vi "Mysql data reader Scalar string.vi"(8 "error in (no error)":errorcluster, 11 ".NET Refnum in":refnum<k24>) -> (0 "error out":errorcluster, 3 "GetString":string)   [LabVIEW 2020, in "mysql.lvlib" / "mysql.lvclass"]
uses:
  mysql.lvclass
  MySql.Data
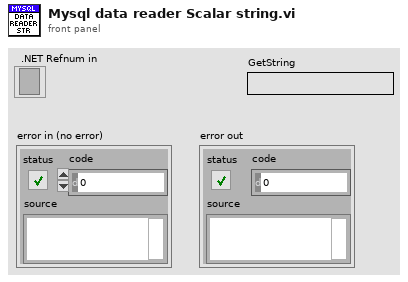
[diagram p1: front panel]
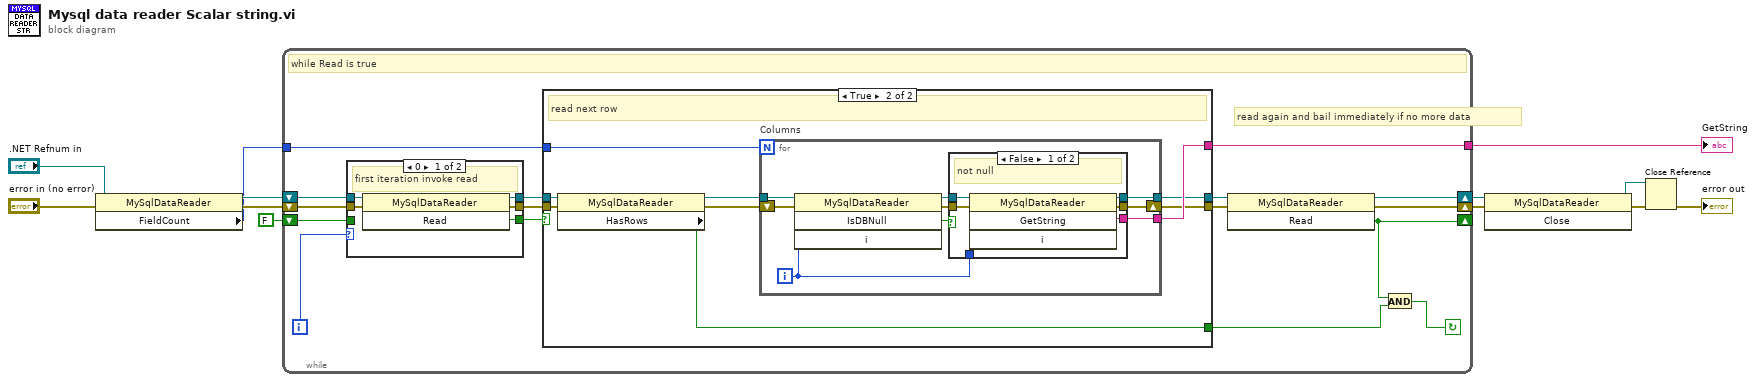
[diagram p0: block diagram]
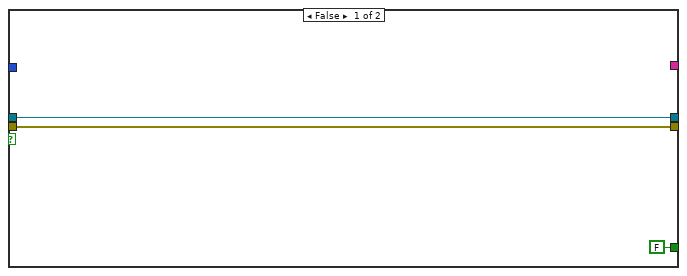
[diagram p3: hidden frame]
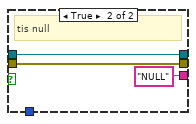
[diagram p4: hidden frame]
diagram:
  n1 = property class="MySqlDataReader"(reference=".NET Refnum in", error in="error in (no error)") -> (reference out=w8:refnum<k24>, error out=w7:errorcluster, "FieldCount"=w4:i32)
  n2 = while {
    tunnel: w4 -> [w28]
    tunnel: [w27] -> w5
    shift-right: [w21] -> w10
    shift-left: w7 -> [w26]
    shift-right: [w19] -> w9
    shift-left: w8 -> [w24]
    shift-right: [w14] -> _
    shift-left: FALSE ("Read") -> [w13]
    i -> [w15]
    stop <- w17 continue-if-true
    # "read again and bail immediately if no more data"
    # "while Read is true"
    n3 = case shown="0" w15 {
      tunnel: w26 -> [w33 w35]
      tunnel: [w32 w35] -> w25
      tunnel: w24 -> [w31 w36]
      tunnel: [w30 w36] -> w23
      tunnel: [w29 w34] -> w22
      tunnel: w13 -> [_ w34]
      frame 0 {
        # "first iteration invoke read"
        n4 = invoke class="MySqlDataReader" method="Read"(reference=w31, error in=w33) -> (reference out=w30:refnum<k24>, error out=w32:errorcluster, "Read"=w29:bool)  [unwired: 1 in]
      }
      frame 1.., Default {
        # "read after for other iterations"
      }
    }
    n5 = case shown="True" w22 {
      tunnel: w28 -> [_ w48]
      tunnel: [_ w47] -> w27
      tunnel: w25 -> [w38 w46]
      tunnel: w23 -> [w39 w45]
      tunnel: [w39 w44] -> w18
      tunnel: [w38 w40] -> w20
      tunnel: [FALSE ("HasRows") w41] -> w16
      frame False {
      }
      frame True {
        # "read next row"
        n6 = property class="MySqlDataReader"(reference=w45, error in=w46) -> (reference out=w43:refnum<k24>, error out=w42:errorcluster, "HasRows"=w41:bool)
        n7 = for "Columns" {
          N: w48 -> [_]
          tunnel: w43 -> [w52]
          shift-right: [w57] -> w40
          shift-left: w42 -> [w53]
          tunnel: [w56] -> w47
          tunnel: [w55] -> w44
          i -> [w54]
          n8 = invoke class="MySqlDataReader" method="IsDBNull"(reference=w52, error in=w53, "i"=w54) -> (reference out=w51:refnum<k24>, error out=w50:errorcluster, "IsDBNull"=w49:bool)  [unwired: 1 in, 1 out]
          n9 = case shown="False" w49 {
            tunnel: [w63 w65] -> w57
            tunnel: [w62 "NULL" ("GetString")] -> w56
            tunnel: [w61 w66] -> w55
            tunnel: w54 -> [w60 _]
            tunnel: w51 -> [w59 w66]
            tunnel: w50 -> [w58 w65]
            frame False {
              # "not null"
              n10 = invoke class="MySqlDataReader" method="GetString"(reference=w59, error in=w58, "i"=w60) -> (reference out=w61:refnum<k24>, error out=w63:errorcluster, "GetString"=w62:string)  [unwired: 1 in, 1 out]
            }
            frame True {
              # "tis null"
            }
          }
        }
      }
    }
    n11 = invoke class="MySqlDataReader" method="Read"(reference=w18, error in=w20) -> (reference out=w19:refnum<k24>, error out=w21:errorcluster, "Read"=w14:bool)  [unwired: 1 in]
    n12 = And(x=w14, y=w16) -> (x .and. y?=w17:bool)
  }
  "GetString" <- w5
  n13 = invoke class="MySqlDataReader" method="Close"(reference=w9, error in=w10) -> (reference out=w12:refnum<k24>, error out=w11:errorcluster)  [unwired: 1 in, 1 out]
  n14 = Close Reference(reference=w12, error in (no error)=w11) -> (error out=→"error out":errorcluster)
